vi "ex_getFileFormat.vi"(11 "Reference":T1) -> (3 "storage_format":enum32{"lvm", "tdm", "tdms", "xlsx"}(ring))   [LabVIEW 2017]
uses:
  <vilib>/express/express shared/propPageData.ctl
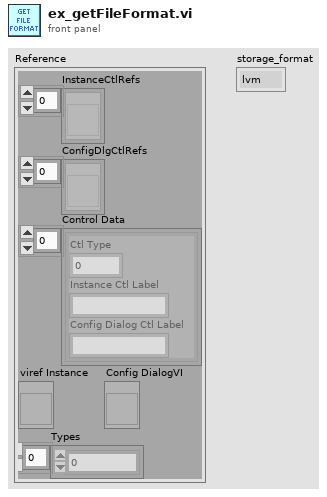
[diagram p1: front panel]
types:
  T1 = typedef "propPageData.ctl" = cluster{"InstanceCtlRefs":refnum<vi>[], "ConfigDlgCtlRefs":refnum<vi>[], "Control Data":cluster{"Ctl Type":u16, "Instance Ctl Label":string, "Config Dialog Ctl Label":string}[], "viref Instance":refnum<vi>, "Types":i32[], "Config DialogVI":refnum<vi>}
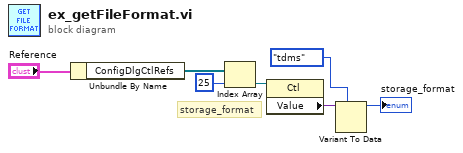
[diagram p0: block diagram]
diagram:
  # "storage_format"
  n1 = Unbundle By Name("Reference") -> ("ConfigDlgCtlRefs"=w3:refnum<vi>[])
  n2 = Index Array(array=w3, index=25) -> (element=w1:refnum<vi>)
  n3 = property class="Ctl"(reference=w1) -> ("Value"=w5:variant)  [unwired: 1 in, 2 out]
  n4 = Variant To Data(type=enum32{"lvm", "tdm", "tdms", "xlsx"}."tdms" ("storage_format"), Variant=w5) -> (data=→"storage_format":enum32{"lvm", "tdm", "tdms", "xlsx"})  [unwired: 1 in, 1 out]
